vi "sub_appcomm_data.vi"() -> (3 "str4app_out":string)   [LabVIEW 2019]
uses:
  Ctrl/pid-status.ctl
  Ctrl/pid-in-params.ctl
panel:
  out "time":string
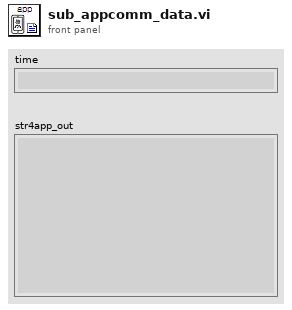
[diagram p1: front panel]
types:
  T1 = typedef "pid-in-params.ctl" = enum16{"read", "write"}
  T2 = typedef "pid-status.ctl" = enum16{"read", "wirte pid dt", "wirte pid output"}
  T3 = cluster{"deg_agv-lookahead":dbl, "deg_waypoint":dbl, "deg_gap":dbl, "deg_target":dbl, "pid output":dbl, "distance-gap_out":dbl}
  T4 = cluster{"progress_curr":dbl, "progress_all":dbl, "distance_left":dbl, "distance_all":dbl}
  T5 = cluster{"System Feedback":cluster{"system state":string, "Control Mode":u8, "Battery Voltage":dbl, "error code High":u8, "error code Low":u8}, "Motion Feedback":cluster{"Linear Velocity (m/s)":dbl, "Angular Velocity (rad/s)":dbl}}
  T6 = cluster{"Linear Velocity (m/s)":dbl, "Angular Velocity (rad/s)":dbl}
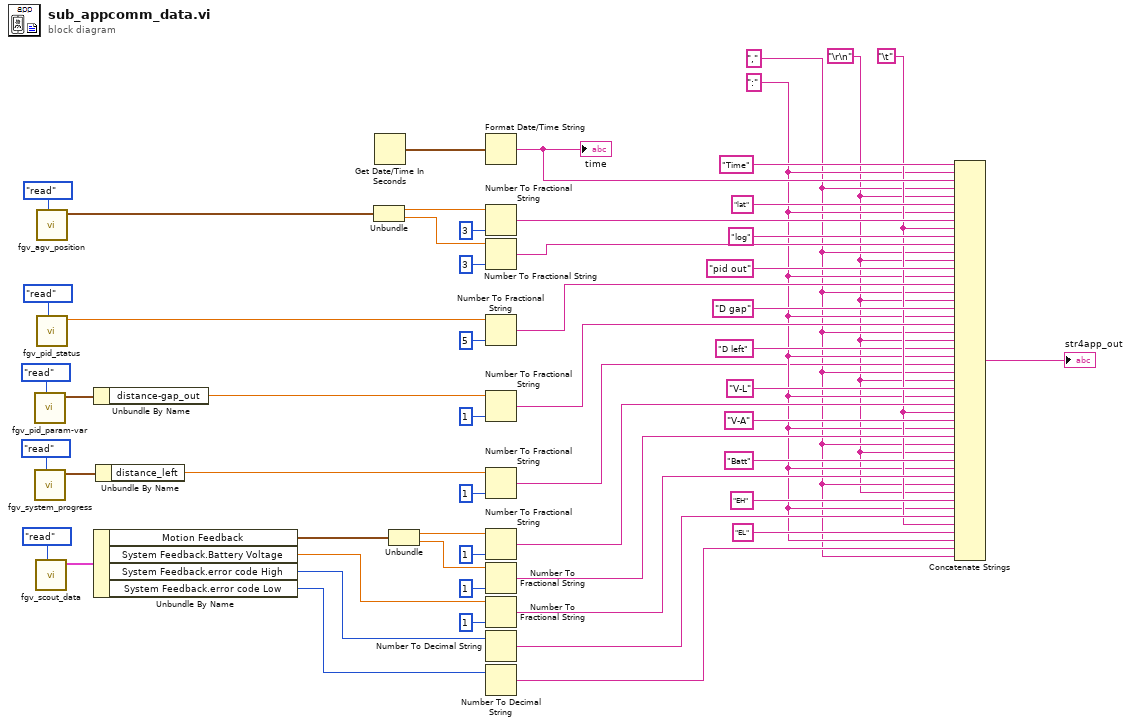
[diagram p0: block diagram]
diagram:
  w10 = "\t"
  w1 = "\r\n"
  w2 = "," ("문자열")
  w4 = ":" ("문자열")
  n1 = call "fgv_pid_param-var.vi"("cmd"=pid-in-params."read") -> ("pid-var_output"=w43:T3)  [unwired: 10 in]
  n2 = call "fgv_system_progress.vi"("cmd"=enum16{"read", "write"}."read") -> ("progress status out"=w8:T4)  [unwired: 10 in]
  n3 = call "fgv_scout_data.vi"("cmd"=enum16{"write", "read"}."read") -> ("agv data out"=w37:T5)  [unwired: 10 in]
  n4 = call "fgv_agv_position.vi"("cmd"=enum16{"write", "read"}."read") -> ("latlong out"=w55:cluster{dbl, dbl})  [unwired: 8 in, 2 out]
  n5 = call "fgv_pid_status.vi"("cmd"=pid-status."read") -> ("pid output"=w47:dbl)  [unwired: 8 in, 2 out]
  n6 = Unbundle By Name(w43) -> ("distance-gap_out"=w42:dbl)
  n7 = Unbundle By Name(w37) -> ("Motion Feedback"=w34:T6, "System Feedback.Battery Voltage"=w24:dbl, "System Feedback.error code High"=w30:u8, "System Feedback.error code Low"=w29:u8)
  n8 = Unbundle By Name(w8) -> ("distance_left"=w6:dbl)
  n9 = Unbundle(w55) -> (w54:dbl, w53:dbl)
  n10 = Get Date/Time In Seconds() -> (seconds since 1Jan1904=w21:timestamp)
  n11 = Unbundle(w34) -> ("Linear Velocity (m/s)"=w35:dbl, "Angular Velocity (rad/s)"=w36:dbl)
  n12 = Format Date/Time String(seconds (now)=w21) -> (date/time string=w20:string)  [unwired: 2 in]
  "time" <- w20
  n13 = Number To Fractional String(number=w54, precision (6)=i16 3 ("정밀도(6)")) -> (F-format string=w52:string)  [unwired: 2 in]
  n14 = Number To Fractional String(number=w53, precision (6)=i16 3 ("정밀도(6)")) -> (F-format string=w49:string)  [unwired: 2 in]
  n15 = Number To Fractional String(number=w47, precision (6)=i16 5 ("정밀도(6)")) -> (F-format string=w45:string)  [unwired: 2 in]
  n16 = Number To Fractional String(number=w42, precision (6)=i16 1 ("정밀도(6)")) -> (F-format string=w40:string)  [unwired: 2 in]
  n17 = Number To Fractional String(number=w6, precision (6)=i16 1 ("정밀도(6)")) -> (F-format string=w3:string)  [unwired: 2 in]
  n18 = Number To Fractional String(number=w35, precision (6)=i16 1 ("정밀도(6)")) -> (F-format string=w32:string)  [unwired: 2 in]
  n19 = Number To Fractional String(number=w36, precision (6)=i16 1 ("정밀도(6)")) -> (F-format string=w11:string)  [unwired: 2 in]
  n20 = Number To Fractional String(number=w24, precision (6)=i16 1 ("정밀도(6)")) -> (F-format string=w22:string)  [unwired: 2 in]
  n21 = Number To Decimal String(number=w30) -> (decimal integer string=w27:string)  [unwired: 1 in]
  n22 = Number To Decimal String(number=w29) -> (decimal integer string=w25:string)  [unwired: 1 in]
  n23 = Concatenate Strings("Time" ("문자열"), w4, w20, w2, w1, "lat" ("문자열"), w4, w52, w10, "log" ("문자열"), w49, w2, w1, "pid out" ("문자열"), w4, w45, w2, w1, "D gap" ("문자열"), w4, w40, w2, w1, "D left" ("문자열"), w4, w3, w2, w1, "V-L" ("문자열"), w4, w32, w10, "V-A" ("문자열"), w4, w11, w2, w1, "Batt" ("문자열"), w4, w22, w2, w1, "EH" ("문자열"), w4, w27, w10, "EL" ("문자열"), w4, w25, w2) -> (→"str4app_out":string)
